vi "Kinesis - KIM101 - Set Jog.vi"() -> ()   [LabVIEW 2017]
uses:
  D:/upwork/Laser Measurement Tool/Laser/tests/KIM101/Thorlabs.MotionControl.Controls.dll
  tests/KIM101/Thorlabs.MotionControl.Controls.dll
  D:/upwork/Laser Measurement Tool/Laser/tests/KIM101/Thorlabs.MotionControl.KCube.InertialMotorCLI.dll
  tests/KIM101/Thorlabs.MotionControl.KCube.InertialMotorCLI.dll
panel:
  in  "direction 2":i32(ring)=1 items=["Increase"=1, "Decrease"=2]
  in  "MOVE":bool
  in  "?":T1={"JogAcceleration"=10000, "JogStepFwd"=100, "JogMode"=2, "JogRate"=500, "JogStepRev"=100} {"JogMode" items=["Continuous"=1, "Step"=2]}
  in  "channel":i32(ring)=1 items=["Channel1"=1, "Channel2"=2, "Channel3"=3, "Channel4"=4]
  in  "SET MOVE PARAMETERS":bool
  in  "Serial Number":string="97000001"
  in  "Zero Channels":bool
  in  "?":bool
  in  "KCubeInertialMotorControl":refnum<k24>(container)
  # "Notes:"
  # "- Ensure that the appropriate .DLLs are copied into your Project Folder. Check that the correct bit type are used depending on your version of LabVIEW\ni.e. 32-bit or 64-bit.\n\n\n\n\n\n\n\n\n\n\n\n\n\n\n- Open the example VI through the LabVIEW Project Explorer to correctly load the User Interface from Thorlabs.MotionControl.Controls.dll."
  # "Thorlabs Hardware: KIM101 - K-Cube Inertial Motor Controller\nhttps://www.thorlabs.com/newgrouppage9.cfm?objectgroup_id=9790&pn=KIM101#9791"
  # "This VI will enable you to run the Kinesis Device panel for the KIM101 Intertial Motor Controller. \nYou will also be able to set Jog Parameters & toggle the Jog Mode, as well as assert control to a particular channel.\n\nInstructions:\n1. Connect your KIM101 device to your PC via USB & power your device. See the product manual for details of device setup\nhttps://www.thorlabs.com/thorproduct.cfm?partnumber=KIM101 \n2. Enter the serial number of the controller into the SerialNumber box below.\n3. Run the VI from the LabVIEW Toolbar.\n6. To end the program, click 'END'."
  # "Example Image of .NET Controller - VI opened via Project Explorer/ not opened via Project Explorer"
  # "VI Not Opened via Project Explorer"
  # "VI Opened via Project Explorer"
  # "- To explore the range of methods available, please visit the .NET API, included with your Kinesis software.\n\n- For tips on building your own VIs with Thorlabs Motion Control Hardware, please see our LabVIEW Guide here.\nhttps://www.thorlabs.com/newgrouppage9.cfm?objectgroup_id=10285"
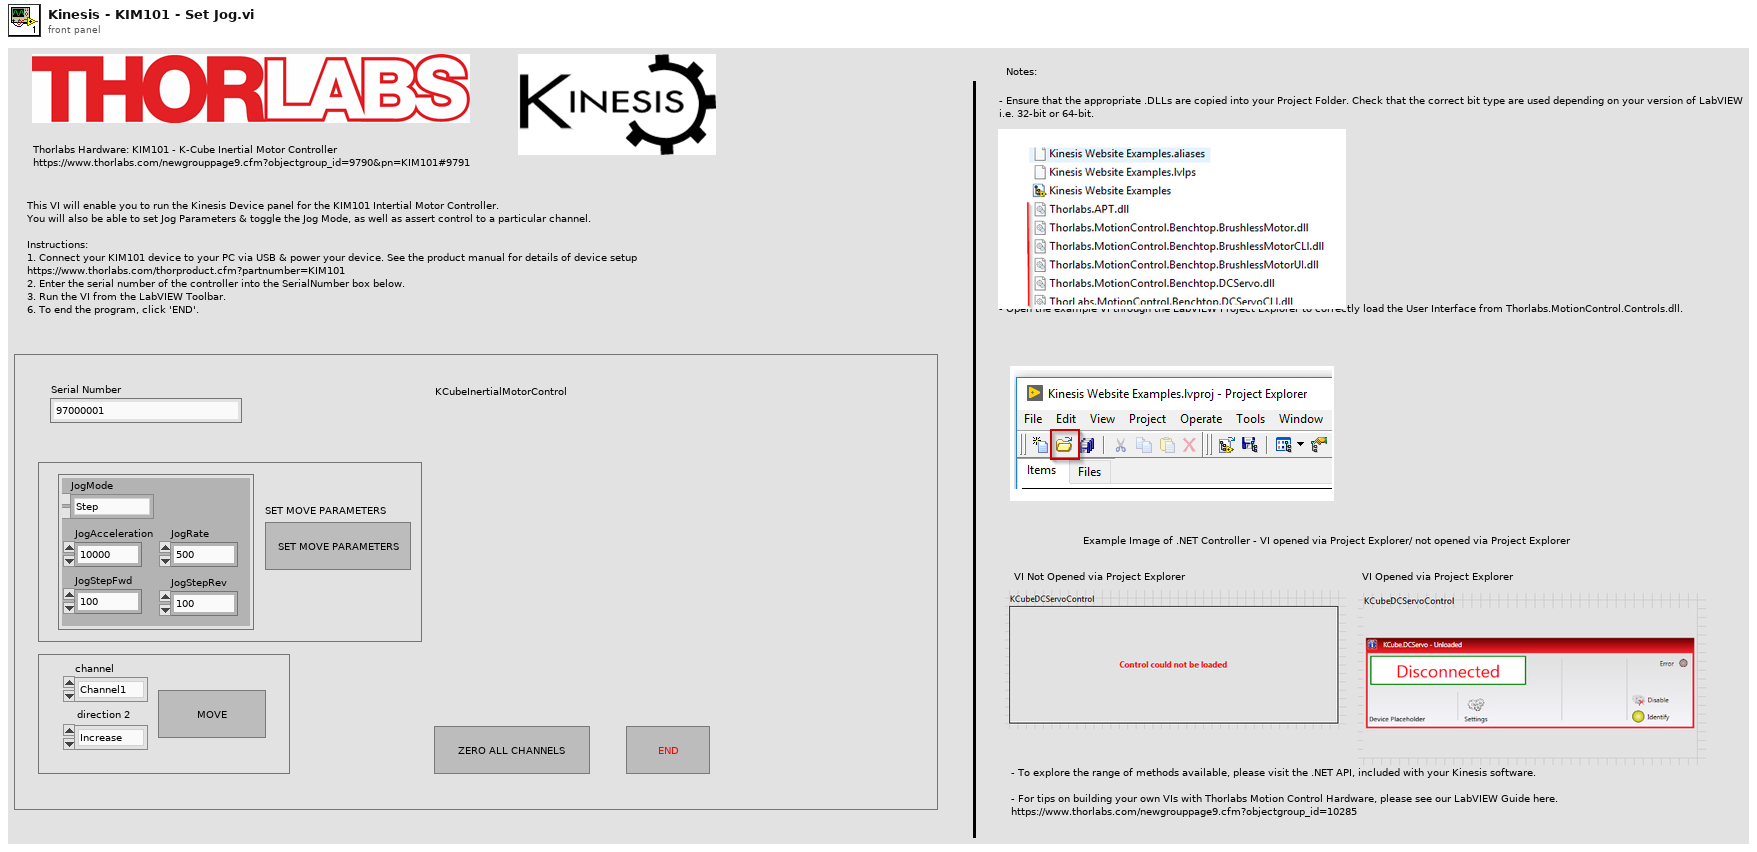
[diagram p1: front panel]
types:
  T1 = cluster{"JogAcceleration":i32, "JogStepFwd":i32, "JogMode":i32, "JogRate":i32, "JogStepRev":i32}
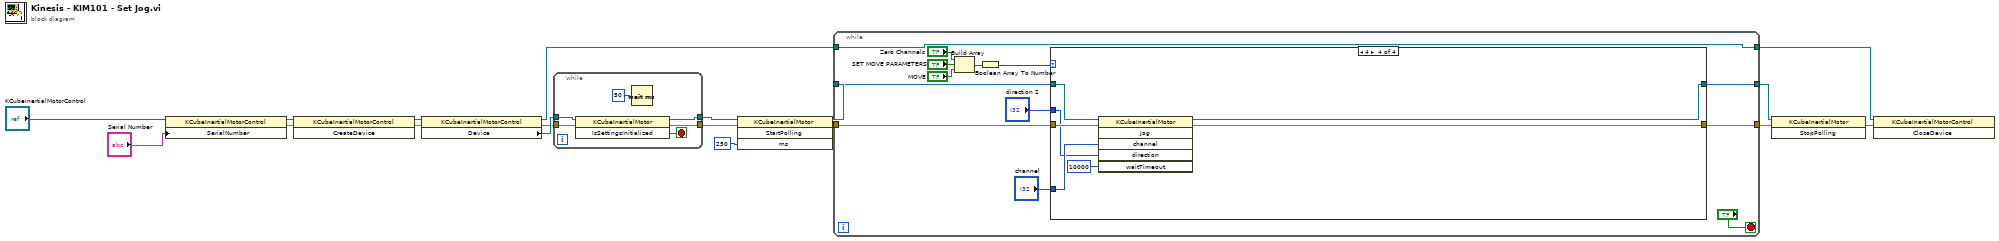
[diagram p0: block diagram]
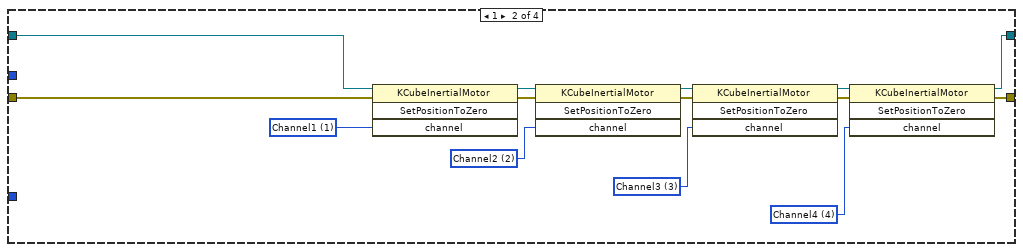
[diagram p3: hidden frame]
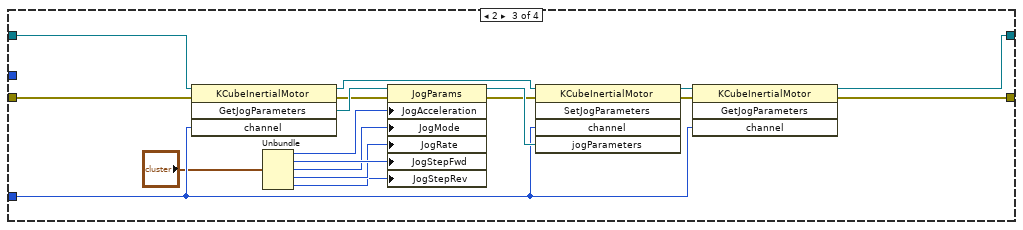
[diagram p4: hidden frame]
diagram:
  n1 = property class="KCubeInertialMotorControl"(reference="KCubeInertialMotorControl", "SerialNumber"="Serial Number") -> (reference out=w17:refnum<k24>, error out=w5:errorcluster)  [unwired: 1 in]
  n2 = invoke class="KCubeInertialMotorControl" method="CreateDevice"(reference=w17, error in=w5) -> (reference out=w15:refnum<k24>, error out=w16:errorcluster)  [unwired: 1 in, 1 out]
  n3 = property class="KCubeInertialMotorControl"(reference=w15, error in=w16) -> (reference out=w3:refnum<k24>, error out=w9:errorcluster, "Device"=w14:refnum<k24>)
  n4 = while {
    tunnel: w14 -> [w24]
    tunnel: [w22] -> w13
    tunnel: w9 -> [w20]
    tunnel: [w19] -> w8
    stop <- w23 stop-if-true
    n5 = invoke class="KCubeInertialMotor" method="IsSettingsInitialized"(reference=w24, error in=w20) -> (reference out=w22:refnum<k24>, error out=w19:errorcluster, "IsSettingsInitialized"=w23:bool)  [unwired: 1 in]
    n6 = Wait (ms)(milliseconds to wait=u32 50) -> ()  [unwired: 1 out]
  }
  n7 = invoke class="KCubeInertialMotor" method="StartPolling"(reference=w13, error in=w8, "ms"=250) -> (reference out=w11:refnum<k24>, error out=w7:errorcluster)  [unwired: 1 in, 2 out]
  n8 = while {
    tunnel: [w34] -> w10
    tunnel: w11 -> [w33]
    tunnel: w7 -> [w32]
    tunnel: [w31] -> w6
    tunnel: [w25] -> w2
    tunnel: w3 -> [w25]
    stop <- "?" stop-if-true
    n9 = Build Array("Zero Channels", "SET MOVE PARAMETERS", "MOVE") -> (w36:bool[])
    n10 = Boolean Array To Number(Boolean array=w36) -> (number=w35:u32)
    n11 = case shown="4" w35 {
      tunnel: [w39 w45 w59 w75] -> w34
      tunnel: w33 -> [w39 w49 w71 w78]
      tunnel: w32 -> [w38 w44 w57 w77]
      tunnel: [w38 w40 w58 w76] -> w31
      tunnel: "channel" -> [_ _ w67 w74]
      tunnel: "direction 2" -> [_ _ _ w73]
      frame 0, Default {
      }
      frame 1 {
        w50 = 4 items=["Channel1"=1, "Channel2"=2, "Channel3"=3, "Channel4"=4] ("channel")
        w51 = 1 items=["Channel1"=1, "Channel2"=2, "Channel3"=3, "Channel4"=4] ("channel")
        w52 = 2 items=["Channel1"=1, "Channel2"=2, "Channel3"=3, "Channel4"=4] ("channel")
        w53 = 3 items=["Channel1"=1, "Channel2"=2, "Channel3"=3, "Channel4"=4] ("channel")
        n12 = invoke class="KCubeInertialMotor" method="SetPositionToZero"(reference=w49, error in=w44, "channel"=w51) -> (reference out=w48:refnum<k24>, error out=w43:errorcluster)  [unwired: 1 in, 2 out]
        n13 = invoke class="KCubeInertialMotor" method="SetPositionToZero"(reference=w48, error in=w43, "channel"=w52) -> (reference out=w47:refnum<k24>, error out=w42:errorcluster)  [unwired: 1 in, 2 out]
        n14 = invoke class="KCubeInertialMotor" method="SetPositionToZero"(reference=w47, error in=w42, "channel"=w53) -> (reference out=w46:refnum<k24>, error out=w41:errorcluster)  [unwired: 1 in, 2 out]
        n15 = invoke class="KCubeInertialMotor" method="SetPositionToZero"(reference=w46, error in=w41, "channel"=w50) -> (reference out=w45:refnum<k24>, error out=w40:errorcluster)  [unwired: 1 in, 2 out]
      }
      frame 2 {
        n16 = invoke class="KCubeInertialMotor" method="GetJogParameters"(reference=w71, error in=w57, "channel"=w67) -> (reference out=w70:refnum<k24>, error out=w56:errorcluster, "GetJogParameters"=w69:refnum<k24>)  [unwired: 1 in, 1 out]
        n17 = Unbundle("?") -> ("JogAcceleration"=w64:i32, "JogStepFwd"=w63:i32, "JogMode"=w62:i32, "JogRate"=w61:i32, "JogStepRev"=w60:i32)
        n18 = property class="JogParams"(reference=w69, error in=w56, "JogAcceleration"=w64, "JogMode"=w62, "JogRate"=w61, "JogStepFwd"=w63, "JogStepRev"=w60) -> (reference out=w68:refnum<k24>, error out=w55:errorcluster)
        n19 = invoke class="KCubeInertialMotor" method="SetJogParameters"(reference=w70, error in=w55, "channel"=w67, "jogParameters"=w68) -> (reference out=w66:refnum<k24>, error out=w54:errorcluster)  [unwired: 1 in, 3 out]
        n20 = invoke class="KCubeInertialMotor" method="GetJogParameters"(reference=w66, error in=w54, "channel"=w67) -> (reference out=w59:refnum<k24>, error out=w58:errorcluster)  [unwired: 1 in, 2 out]
      }
      frame 4 {
        n21 = invoke class="KCubeInertialMotor" method="Jog"(reference=w78, error in=w77, "channel"=w74, "direction"=w73, "waitTimeout"=10000) -> (reference out=w75:refnum<k24>, error out=w76:errorcluster)  [unwired: 1 in, 4 out]
      }
    }
  }
  n22 = invoke class="KCubeInertialMotor" method="StopPolling"(reference=w10, error in=w6) -> (error out=w1:errorcluster)  [unwired: 1 in, 2 out]
  n23 = invoke class="KCubeInertialMotorControl" method="CloseDevice"(reference=w2, error in=w1) -> ()  [unwired: 1 in, 3 out]
